vi "VISA Data Decode.vi"(8 "error in (no error)":errorcluster, 9 "UI Q":refnum<queue>, 10 "Msg":string, 11 "VISA Decode":T1) -> (0 "error out":errorcluster, 3 "VISA Decode out":T1)   [LabVIEW 2015]
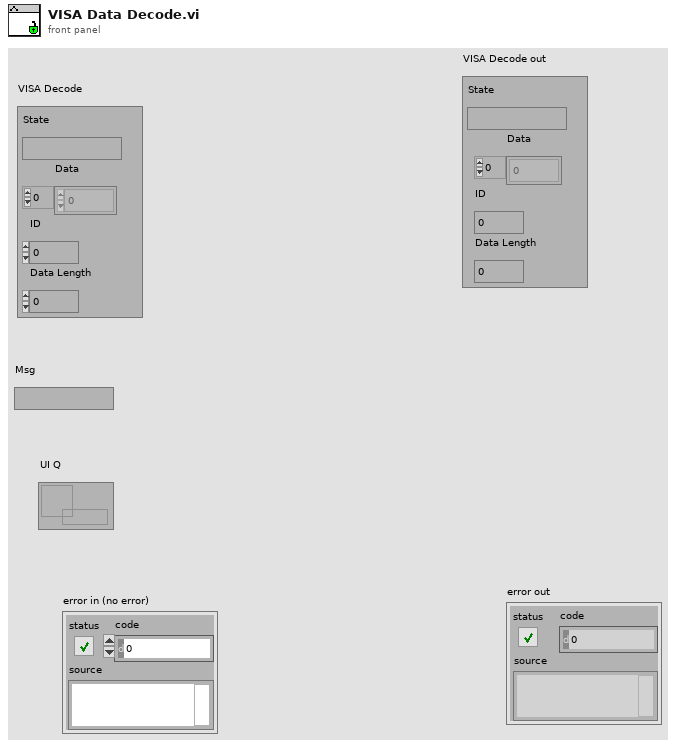
[diagram p1: front panel]
types:
  T1 = cluster{"State":string, "Data":u8[], "ID":u8, "Data Length":i32}
  T2 = cluster{string, "VISA Decode":cluster{"State":string, "Data":u8[], "ID":u8, "Data Length":i32}}
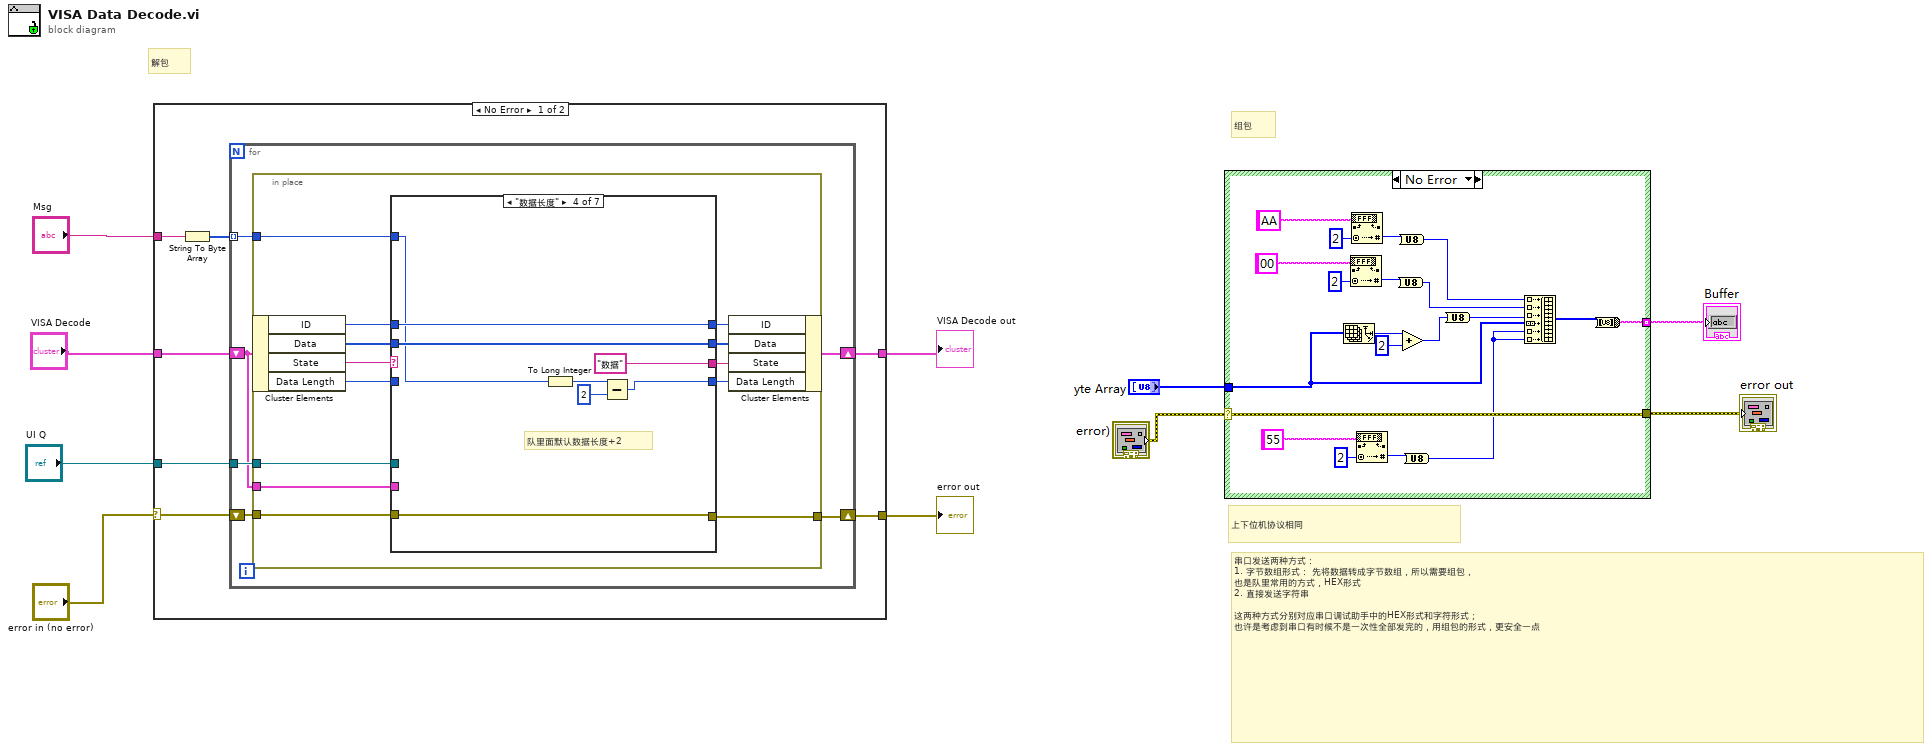
[diagram p0: block diagram]
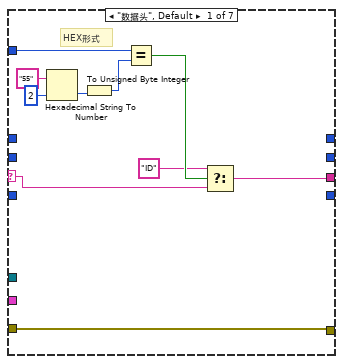
[diagram p2: hidden frame]
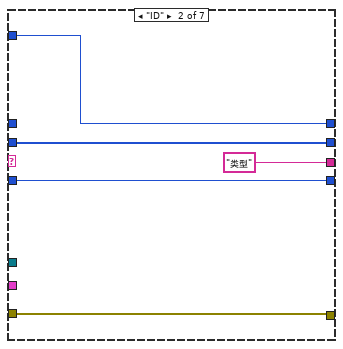
[diagram p3: hidden frame]
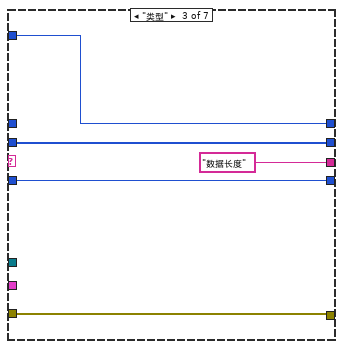
[diagram p4: hidden frame]
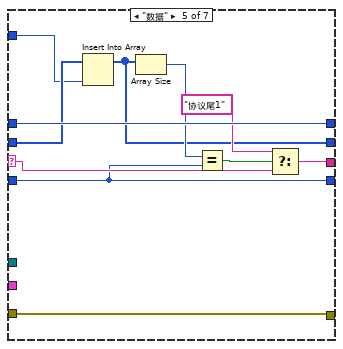
[diagram p5: hidden frame]
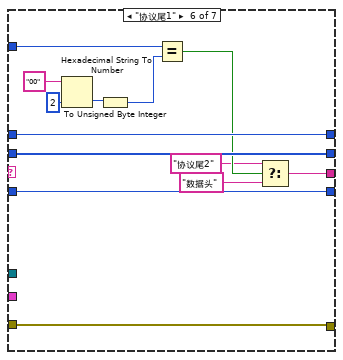
[diagram p6: hidden frame]
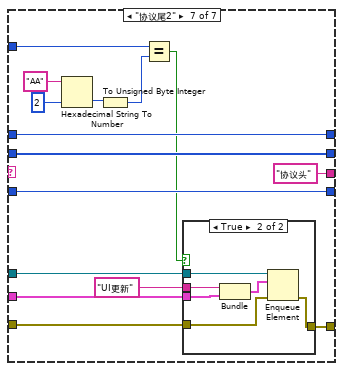
[diagram p7: hidden frame]
diagram:
  # "组包"
  # "解包"
  # "串口发送两种方式：\n1. 字节数组形式： 先将数据转成字节数组，所以需要组包，\n也是队里常用的方式，HEX形式\n2. 直接发送字符串\n\n这两种方式分别对应串口调试助手中的HEX形式和字符形式；\n也许是考虑到串口有时候不是一次性全部发完的，用组包的形式，更安全一点"
  # "上下位机协议相同"
  n1 = case shown="No Error" "error in (no error)" {
    selector: "error in (no error)" -> [w9 w108]
    tunnel: "Msg" -> [w13 _]
    tunnel: "VISA Decode" -> [w11 w107]
    tunnel: "UI Q" -> [w10 _]
    tunnel: [w8 w108] -> w2
    tunnel: [w7 w107] -> w1
    frame No Error {
      n2 = String To Byte Array(string=w13) -> (unsigned byte array=w12:u8[])
      n3 = for {
        tunnel: w12 -> [w19] mode=indexing
        shift-right: [w18] -> w7
        shift-left: w11 -> [w16]
        tunnel: w10 -> [w17]
        shift-right: [w14] -> w8
        shift-left: w9 -> [w15]
        n4 = in-place {
          in-place-border: w19 -> [w32]
          in-place-border: w17 -> [w23]
          in-place-border: w16 -> [w22]
          in-place-border: w15 -> [w21]
          in-place-border: [w20] -> w14
          n5 = in-place-cluster #1(w16) -> ("ID"=w28:u8, "Data"=w27:u8[], "State"=w31:string, "Data Length"=w24:i32)
          n6 = case shown="\"数据长度\"" w31 {
            selector: w31 -> [w36 _ _ _ w65 _ _]
            tunnel: w32 -> [w42 w47 w52 w57 w69 w81 w96]
            tunnel: [w34 "类型" ("t") "数据长度" ("t") "数据" ("t") w66 w75 "协议头" ("f")] -> w30
            tunnel: [_ w47 w52 w60 w71 w84 w99] -> w29
            tunnel: w28 -> [_ _ _ w60 w71 w84 w99]
            tunnel: w27 -> [_ w45 w50 w59 w70 w83 w98]
            tunnel: [_ w45 w50 w59 w63 w83 w98] -> w26
            tunnel: [_ w44 w49 w53 w62 w82 w97] -> w25
            tunnel: w24 -> [_ w44 w49 _ w62 w82 w97]
            tunnel: w23 -> [_ _ _ _ _ _ w89]
            tunnel: w22 -> [_ _ _ _ _ _ w88]
            tunnel: w21 -> [w33 w43 w48 w56 w61 w72 w86]
            tunnel: [w33 w43 w48 w56 w61 w72 w85] -> w20
            frame "数据头", Default {
              # "HEX形式"
              n7 = Hexadecimal String To Number(string="55", default (0uL)=u32 2 ("default (0 U32)")) -> (number=w39:u32)  [unwired: 1 in, 1 out]
              n8 = To Unsigned Byte Integer(number=w39) -> (unsigned 8bit integer=w38:u8)
              n9 = Equal?(x=w42, y=w38) -> (x = y?=w37:bool)
              n10 = Select(t="ID", s=w37, f=w36) -> (s? t:f=w34:string)
            }
            frame "ID" {
            }
            frame "类型" {
            }
            frame "数据长度" {
              # "队里面默认数据长度+2"
              n11 = To Long Integer(number=w57) -> (32bit integer=w55:i32)
              n12 = Subtract(x=w55, y=2) -> (x-y=w53:i32)
            }
            frame "数据" {
              n13 = Insert Into Array(array=w70, new element=w69) -> (w63:u8[])  [unwired: 1 in]
              n14 = Array Size(array=w63) -> (size(s)=w68:i32)
              n15 = Equal?(x=w68, y=w62) -> (x = y?=w67:bool)
              n16 = Select(t="协议尾1", s=w67, f=w65) -> (s? t:f=w66:string)
            }
            frame "协议尾1" {
              n17 = Hexadecimal String To Number(string="00", default (0uL)=u32 2 ("default (0 U32)")) -> (number=w78:u32)  [unwired: 1 in, 1 out]
              n18 = To Unsigned Byte Integer(number=w78) -> (unsigned 8bit integer=w77:u8)
              n19 = Equal?(x=w81, y=w77) -> (x = y?=w76:bool)
              n20 = Select(t="协议尾2", s=w76, f="数据头") -> (s? t:f=w75:string)
            }
            frame "协议尾2" {
              n21 = Hexadecimal String To Number(string="AA", default (0uL)=u32 2 ("default (0 U32)")) -> (number=w93:u32)  [unwired: 1 in, 1 out]
              n22 = To Unsigned Byte Integer(number=w93) -> (unsigned 8bit integer=w92:u8)
              n23 = Equal?(x=w96, y=w92) -> (x = y?=w90:bool)
              n24 = case shown="True" w90 {
                tunnel: w89 -> [_ w106]
                tunnel: w88 -> [_ w105]
                tunnel: "UI更新" -> [_ w103]
                tunnel: w86 -> [w100 w102]
                tunnel: [w100 w101] -> w85
                frame False {
                }
                frame True {
                  n25 = Bundle(w103, "VISA Decode"=w105) -> (w104:T2)  [unwired: 1 in]
                  n26 = Enqueue Element(queue=w106, element=w104, error in (no error)=w102) -> (error out=w101:errorcluster)  [unwired: 1 in, 2 out]
                }
              }
            }
          }
          n27 = in-place-cluster #1("ID"=w29, "Data"=w26, "State"=w30, "Data Length"=w25) -> (w18:T1)
        }
      }
    }
    frame Error {
    }
  }
  "error out" <- w2
  "VISA Decode out" <- w1
